vi "Dryer Status.vi"(0 "Bytes Comm":u8[](array[numeric]), 5 "Fault Cond Detected":bool, 7 "Dryer Status Serial Data In":T1, 9 "Com Port":u8, 11 "Err Count Lim":u32=10) -> (8 "Dryer Status Serial Data Out":T1)   [LabVIEW 2012]
uses:
  Dryer Com Port Info.ctl
  Dryer Status Ctrl.ctl
  Globals Wilt.vi
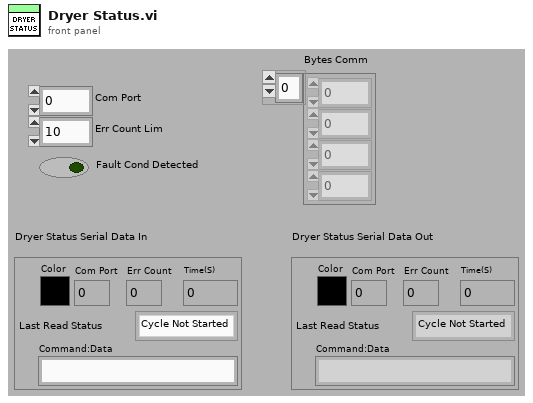
[diagram p1: front panel]
types:
  T1 = typedef "Dryer Com Port Info.ctl" = cluster{"Color":u32, "Last Read Status":T2, "Command:Data":string, "Com Port":u8, "Time(S)":dbl, "Err Count":u32}
  T2 = typedef "Dryer Status Ctrl.ctl" = enum16{"Cycle Not Started", "Cycle Running", "Paused", "Cycle Completed", "Eval Mode Entered", "Err", "Pause (No GEA2)"}
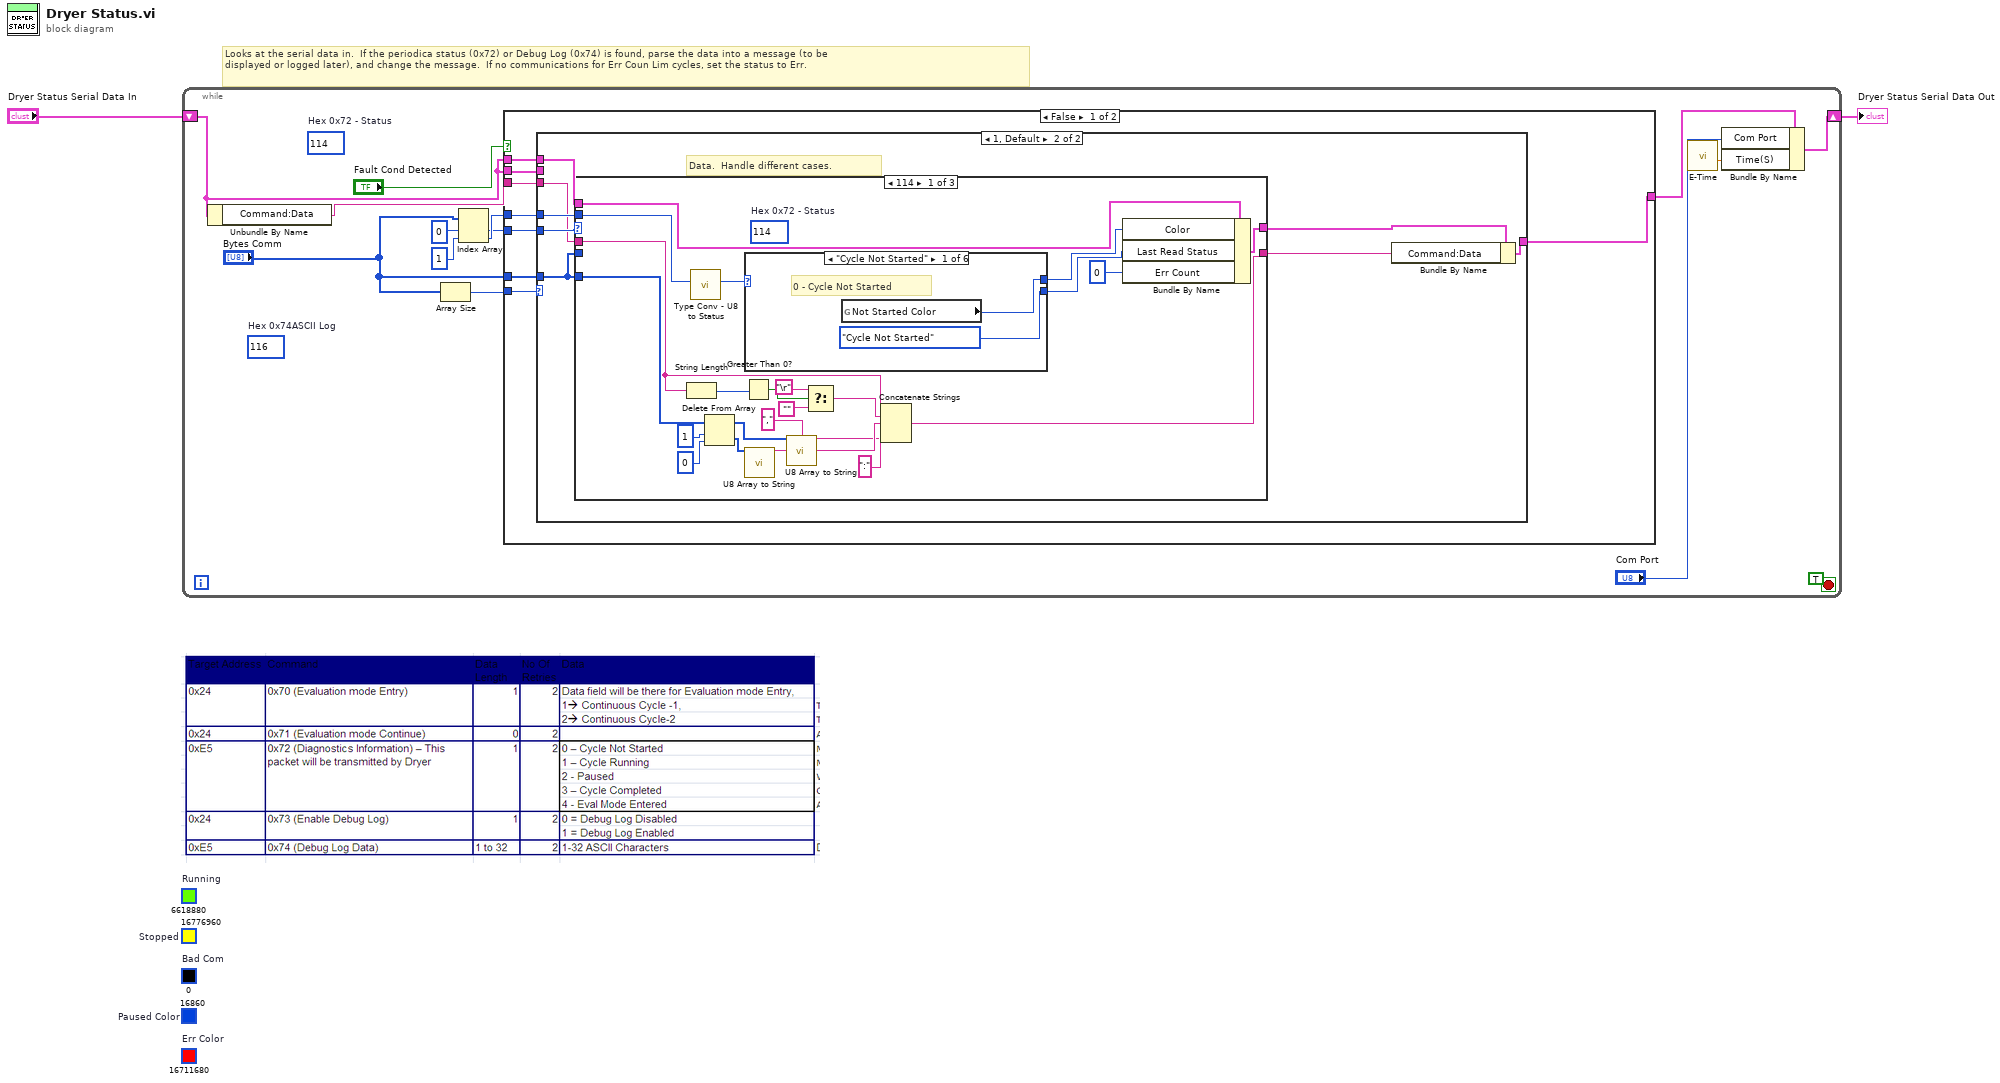
[diagram p0: block diagram]
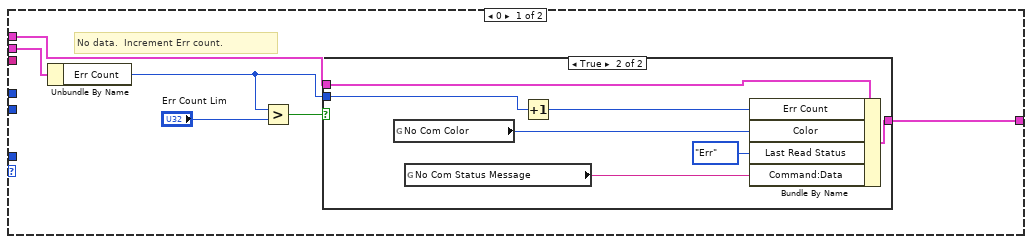
[diagram p2: hidden frame]
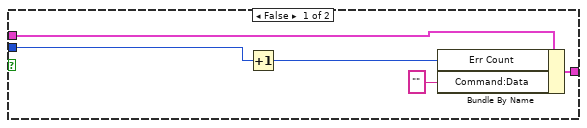
[diagram p3: hidden frame]
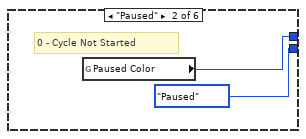
[diagram p4: hidden frame]
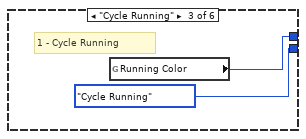
[diagram p5: hidden frame]
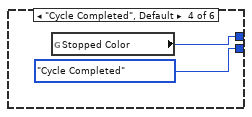
[diagram p6: hidden frame]
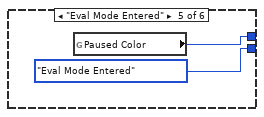
[diagram p7: hidden frame]
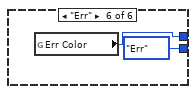
[diagram p8: hidden frame]
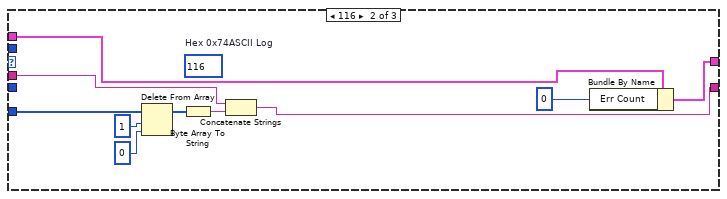
[diagram p9: hidden frame]
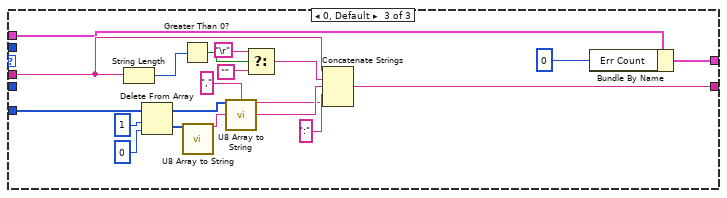
[diagram p10: hidden frame]
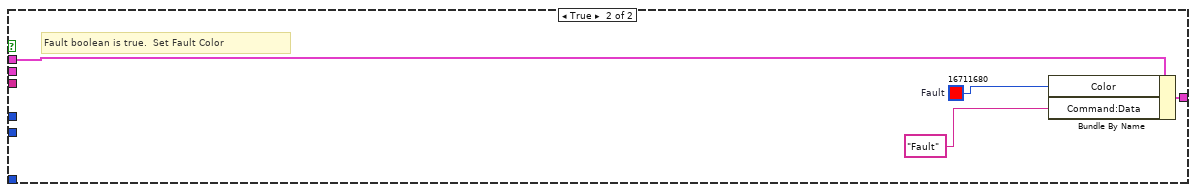
[diagram p11: hidden frame]
diagram:
  (unwired) u32 16711680  # Err Color
  (unwired) u32 16860  # Paused Color
  (unwired) u32 0  # Bad Com
  (unwired) u32 6618880  # Running
  (unwired) u32 16776960  # Stopped
  # "Looks at the serial data in.  If the periodica status (0x72) or Debug Log (0x74) is found, parse the data into a message (to be \ndisplayed or logged later), and change the message.  If no communications for Err Coun Lim cycles, set the status to Err."
  n1 = while {
    shift-right: [w10] -> w1
    shift-left: "Dryer Status Serial Data In" -> [w4]
    stop <- TRUE stop-if-true
    (unwired) 116  # Hex 0x74ASCII Log
    (unwired) 114  # Hex 0x72 - Status
    n2 = Unbundle By Name(w4) -> ("Command:Data"=w3:string)
    n3 = Array Size(array="Bytes Comm") -> (size(s)=w15:i32)
    n4 = Index Array(array="Bytes Comm", index #1=0 ("index"), index #2=1 ("index")) -> (element #1=w9:u8, element #2=w12:u8)
    n5 = case shown="False" "Fault Cond Detected" {
      tunnel: w15 -> [w24 _]
      tunnel: w12 -> [w23 _]
      tunnel: w9 -> [w22 _]
      tunnel: w4 -> [w21 w115]
      tunnel: [w20 w116] -> w8
      tunnel: "Bytes Comm" -> [w19 _]
      tunnel: w4 -> [w18 _]
      tunnel: w3 -> [w17 _]
      frame False {
        n6 = case shown="1, Default" w24 {
          tunnel: w23 -> [_ w47]
          tunnel: w22 -> [_ w46]
          tunnel: w21 -> [w30 w50]
          tunnel: [w29 w48] -> w20
          tunnel: w19 -> [_ w44]
          tunnel: w18 -> [w28 _]
          tunnel: w17 -> [_ w45]
          frame 0 {
            # "No data.  Increment Err count."
            n7 = Unbundle By Name(w28) -> ("Err Count"=w27:u32)
            n8 = Greater?(x=w27, y="Err Count Lim") -> (0:w25:bool)
            n9 = case shown="True" w25 {
              tunnel: w30 -> [w35 w42]
              tunnel: [w34 w41] -> w29
              tunnel: w27 -> [w32 w39]
              frame False {
                n10 = Increment(x=w32) -> (x+1=w33:u32)
                n11 = Bundle By Name(cluster=w35, "Err Count"=w33, "Command:Data"="") -> (w34:T1)
              }
              frame True {
                n12 = global read "Globals Wilt.vi" "No Com Color"() -> (w36:u32)
                n13 = global read "Globals Wilt.vi" "No Com Status Message"() -> (w37:string)
                n14 = Increment(x=w39) -> (x+1=w38:u32)
                n15 = Bundle By Name(cluster=w42, "Err Count"=w38, "Color"=w36, "Last Read Status"=Dryer_Status_Ctrl."Err" ("Status"), "Command:Data"=w37) -> (w41:T1)
              }
            }
          }
          frame 1, Default {
            # "Data.  Handle different cases."
            n16 = case shown="114" w46 {
              tunnel: w47 -> [w52 _ _]
              tunnel: w50 -> [w73 w88 w97]
              tunnel: [w72 w87 w96] -> w49
              tunnel: w44 -> [_ _ _]
              tunnel: w45 -> [w56 w91 w101]
              tunnel: w44 -> [w57 w92 w102]
              tunnel: [w54 w89 w99] -> w43
              frame 114 {
                (unwired) 114  # Hex 0x72 - Status
                n17 = String Length(string=w56) -> (length=w64:i32)
                n18 = call "Type Conv - U8 to Status.vi"("Byte Val"=w52) -> ("Status"=w53:T2)  [unwired: 10 in]
                n19 = Delete From Array(array=w57, length=1, index=0) -> (deleted portion=w58:u8[], array with subset deleted=w55:u8[])
                n20 = Greater Than 0?(x=w64) -> (x > 0?=w65:bool)
                n21 = case shown="\"Cycle Not Started\"" w53 {
                  tunnel: [w74 w77 w79 w80 w83 w85] -> w70
                  tunnel: [Dryer_Status_Ctrl."Cycle Not Started" ("Status") Dryer_Status_Ctrl."Paused" ("Status") Dryer_Status_Ctrl."Cycle Running" ("Status") Dryer_Status_Ctrl."Cycle Completed" ("Status") Dryer_Status_Ctrl."Eval Mode Entered" ("Status") Dryer_Status_Ctrl."Err" ("Status")] -> w71
                  frame "Cycle Not Started" {
                    # "0 - Cycle Not Started"
                    n22 = global read "Globals Wilt.vi" "Not Started Color"() -> (w74:u32)
                  }
                  frame "Paused" {
                    # "0 - Cycle Not Started"
                    n23 = global read "Globals Wilt.vi" "Paused Color"() -> (w77:u32)
                  }
                  frame "Cycle Running" {
                    # "1 - Cycle Running"
                    n24 = global read "Globals Wilt.vi" "Running Color"() -> (w79:u32)
                  }
                  frame "Cycle Completed", Default {
                    n25 = global read "Globals Wilt.vi" "Stopped Color"() -> (w80:u32)
                  }
                  frame "Eval Mode Entered" {
                    n26 = global read "Globals Wilt.vi" "Paused Color"() -> (w83:u32)
                  }
                  frame "Err" {
                    n27 = global read "Globals Wilt.vi" "Err Color"() -> (w85:u32)
                  }
                }
                n28 = call "U8 Array to String.vi"("U8 Data"=w58) -> ("String"=w61:string)  [unwired: 14 in]
                n29 = call "U8 Array to String.vi"("U8 Data"=w55, "Delimiter(_)"=",") -> ("String"=w59:string)  [unwired: 13 in]
                n30 = Select(t="\r", s=w65, f="") -> (s? t:f=w68:string)
                n31 = Concatenate Strings(w56, w68, w61, ":" ("string"), w59) -> (w54:string)
                n32 = Bundle By Name(cluster=w73, "Color"=w70, "Last Read Status"=w71, "Err Count"=u32 0) -> (w72:T1)
              }
              frame 116 {
                (unwired) 116  # Hex 0x74ASCII Log
                n33 = Delete From Array(array=w92, length=1, index=0) -> (array with subset deleted=w90:u8[])  [unwired: 1 out]
                n34 = Byte Array To String(unsigned byte array=w90) -> (string=w93:string)
                n35 = Concatenate Strings(w91, w93) -> (w89:string)
                n36 = Bundle By Name(cluster=w88, "Err Count"=u32 0) -> (w87:T1)
              }
              frame 0, Default {
                n37 = String Length(string=w101) -> (length=w109:i32)
                n38 = Delete From Array(array=w102, length=1, index=0) -> (deleted portion=w103:u8[], array with subset deleted=w100:u8[])
                n39 = Greater Than 0?(x=w109) -> (x > 0?=w110:bool)
                n40 = call "U8 Array to String.vi"("U8 Data"=w103) -> ("String"=w106:string)  [unwired: 14 in]
                n41 = call "U8 Array to String.vi"("U8 Data"=w100, "Delimiter(_)"=",") -> ("String"=w104:string)  [unwired: 13 in]
                n42 = Select(t="\r", s=w110, f="") -> (s? t:f=w113:string)
                n43 = Concatenate Strings(w101, w113, w106, ":" ("string"), w104) -> (w99:string)
                n44 = Bundle By Name(cluster=w97, "Err Count"=u32 0) -> (w96:T1)
              }
            }
            n45 = Bundle By Name(cluster=w49, "Command:Data"=w43) -> (w48:T1)
          }
        }
      }
      frame True {
        w118 = u32 16711680  # Fault
        # "Fault boolean is true.  Set Fault Color"
        n46 = Bundle By Name(cluster=w115, "Color"=w118, "Command:Data"="Fault" ("Status")) -> (w116:T1)
      }
    }
    n47 = call "E-Time.vi"() -> ("Elapsed Time (sec)"=w5:dbl)  [unwired: 9 in, 2 out]
    n48 = Bundle By Name(cluster=w8, "Com Port"="Com Port", "Time(S)"=w5) -> (w10:T1)
  }
  "Dryer Status Serial Data Out" <- w1
